vi "Write FP Type.vi"(8 "error in (no error)":errorcluster, 10 "FP Type":T1=enum."CF", 11 "Inst.FP in":refnum<class "Inst.FP.lvclass">) -> (0 "error out":errorcluster, 3 "Inst.FP out":refnum<class "Inst.FP.lvclass">)   [LabVIEW 2019, in "Inst.FP.lvclass"]
uses:
  Inst.FP.lvclass
  Typedefs/Inst.FP.Type--Enum.ctl
  Inst.FP.lvclass/Inst.FP.ctl
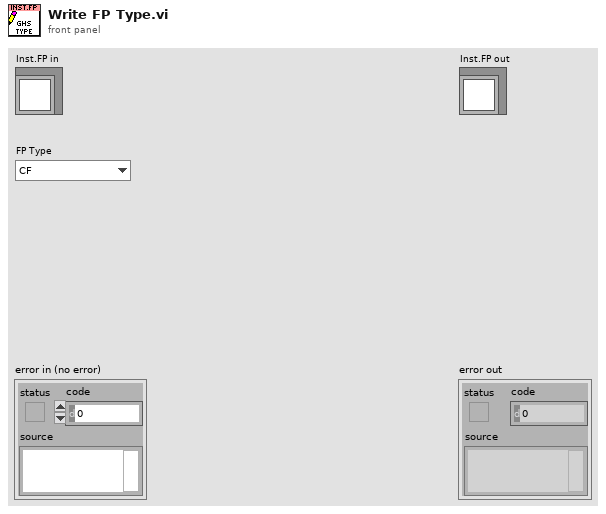
[diagram p1: front panel]
types:
  T1 = typedef "Inst.FP.lvclass/Inst.FP.Type--Enum.ctl" = enum32{"Wet", "CF"}
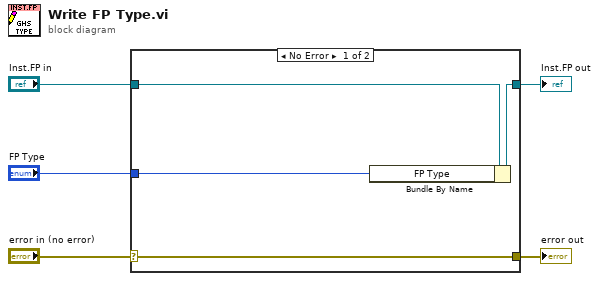
[diagram p0: block diagram]
diagram:
  n1 = case shown="No Error" "error in (no error)" {
    selector: "error in (no error)" -> [w9 w10]
    tunnel: [w9 w10] -> w4
    tunnel: [w7 w11] -> w2
    tunnel: "Inst.FP in" -> [w8 w11]
    tunnel: "FP Type" -> [w6 _]
    frame No Error {
      n2 = Bundle By Name(cluster=w8, "FP Type"=w6) -> (w7:refnum<class "Inst.FP.lvclass">)
    }
    frame Error {
    }
  }
  "error out" <- w4
  "Inst.FP out" <- w2
